vi "GetNumberOfDocs.vi"(8 "error in (no error)":errorcluster, 11 "MongoDB-Collection in":refnum<class "MongoDB-Collection.lvclass">) -> (0 "error out":errorcluster, 2 "GetNumberOfDocs":i64, 3 "MongoDB-Collection out":refnum<class "MongoDB-Collection.lvclass">)   [LabVIEW 2016, in "MongoDB-Collection.lvlib" / "MongoDB-Collection.lvclass"]
uses:
  MongoDB-Collection.lvclass
  D:/Users/blume/Desktop/LV/MongoDB-Driver/MLV DLLs/MongoLabVIEW.dll
  LV/MongoDB-Driver/MLV DLLs/MongoLabVIEW.dll
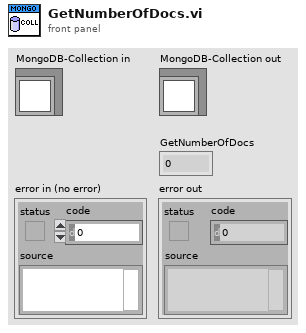
[diagram p1: front panel]
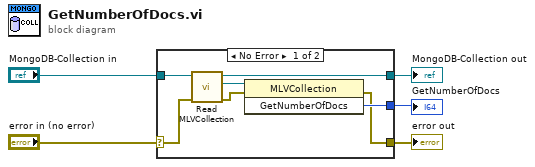
[diagram p0: block diagram]
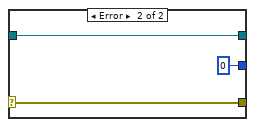
[diagram p2: hidden frame]
diagram:
  n1 = case shown="No Error" "error in (no error)" {
    selector: "error in (no error)" -> [w11 w15]
    tunnel: [w6 w15] -> w4
    tunnel: [w8 w14] -> w2
    tunnel: "MongoDB-Collection in" -> [w12 w14]
    tunnel: [w7 i64 0 ("GetNumberOfDocs")] -> w1
    frame No Error {
      n2 = call "Read MLVCollection.vi"("error in (no error)"=w11, "MongoDB-Collection in"=w12) -> ("error out"=w9:errorcluster, "MLVCollection"=w10:refnum<k24>, "MongoDB-Collection out"=w8:refnum<class "MongoDB-Collection.lvclass">)  [unwired: 7 in]
      n3 = invoke class="MLVCollection" method="GetNumberOfDocs"(reference=w10, error in=w9) -> (error out=w6:errorcluster, "GetNumberOfDocs"=w7:i64)  [unwired: 1 in, 1 out]
    }
    frame Error {
    }
  }
  "error out" <- w4
  "MongoDB-Collection out" <- w2
  "GetNumberOfDocs" <- w1
